vi "get_lin_signal_raw_value.vi"(8 "错误输入（无错误）":errorcluster, 9 "FDatas":T1, 10 "TLINSignal":T2, 11 "路径输入":path) -> (0 "错误输出":errorcluster, 2 "Signal_Value":dbl, 3 "路径输出":path)   [LabVIEW 2014]
uses:
  Typedef/LIN/TLINSignal.ctl
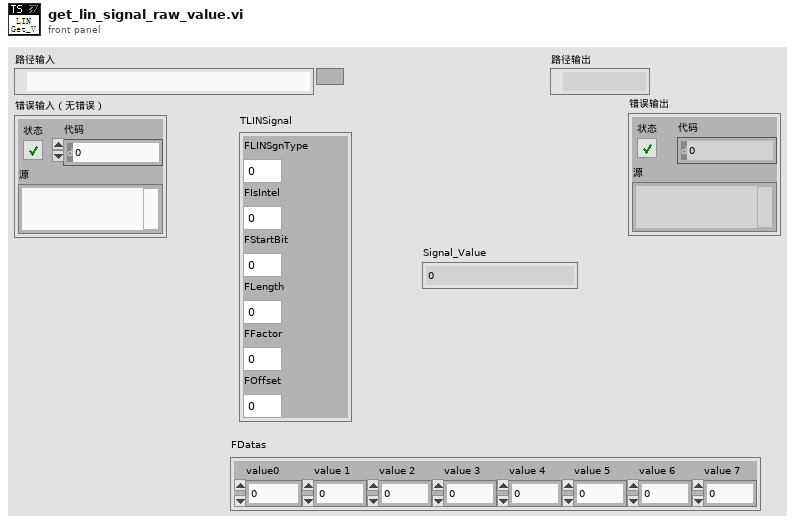
[diagram p1: front panel]
types:
  T1 = cluster{"value0":u8, "value 1":u8, "value 2":u8, "value 3":u8, "value 4":u8, "value 5":u8, "value 6":u8, "value 7":u8}
  T2 = typedef "TLINSignal.ctl" = cluster{"FLINSgnType":u8, "FIsIntel":u8, "FStartBit":i32, "FLength":i32, "FFactor":dbl, "FOffset":dbl}
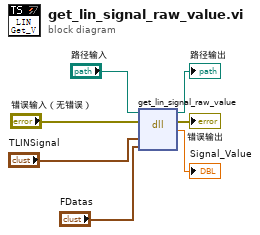
[diagram p0: block diagram]
diagram:
  n1 = dll-call lib="D:/Program Files (x86)/TOSUN/TSMaster/bin/TSMaster.dll" fn="get_lin_signal_raw_value"(path in="路径输入", error in="错误输入（无错误）", "TLINSignal"="TLINSignal", "FDatas"="FDatas") -> (path out=→"路径输出":path, error out=→"错误输出":errorcluster, "Signal_Value"=→"Signal_Value":dbl)  [unwired: 3 in]
